vi "Add Annotation.vi"(8 "error in (no error)":errorcluster, 9 "Style":T1, 10 "Name":string, 11 "FSM.Edge in":refnum<class "FSM.Edge.lvclass">) -> (0 "error out":errorcluster, 2 "Changed?":bool, 3 "FSM.Edge out":refnum<class "FSM.Edge.lvclass">)   [LabVIEW 2015, in "FSM.Edge.lvclass"]
uses:
  FSM.Edge.lvclass
  FSM.Annotation/Annotation Style.ctl
  FSM.Edge.lvclass/FSM.Edge.ctl
  FSM.Annotation/FSM.Annotation.lvclass
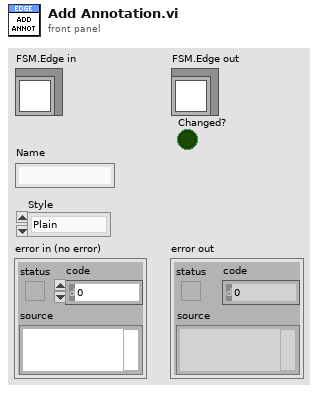
[diagram p1: front panel]
types:
  T1 = typedef "FSM.Annotation.lvclass/Annotation Style.ctl" = enum16{"Plain", "On", "Off", "On-Off"}
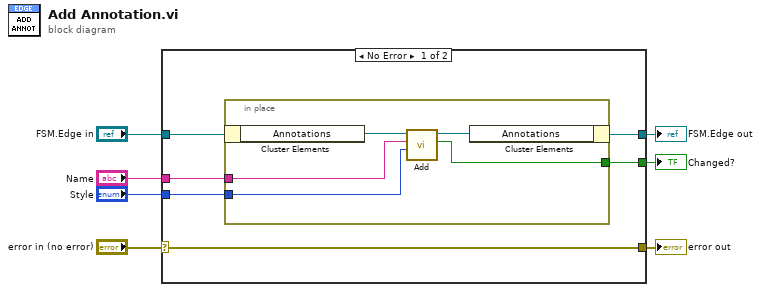
[diagram p0: block diagram]
diagram:
  n1 = case shown="No Error" "error in (no error)" {
    selector: "error in (no error)" -> [w13 w20]
    tunnel: [w13 w20] -> w6
    tunnel: [w9 w19] -> w4
    tunnel: "FSM.Edge in" -> [w10 w19]
    tunnel: "Name" -> [w11 _]
    tunnel: "Style" -> [w12 _]
    tunnel: [w8 _] -> w1
    frame No Error {
      n2 = in-place {
        in-place-border: w12 -> [w15]
        in-place-border: w11 -> [w16]
        in-place-border: [w14] -> w8
        n3 = in-place-cluster #1(w10) -> ("Annotations"=w18:refnum<class "FSM.Annotation.lvclass">)
        n4 = call "Add.vi"("Style"=w15, "Name"=w16, "FSM.Annotation in"=w18) -> ("Changed?"=w14:bool, "FSM.Annotation out"=w17:refnum<class "FSM.Annotation.lvclass">)  [unwired: 6 in, 1 out]
        n5 = in-place-cluster #1("Annotations"=w17) -> (w9:refnum<class "FSM.Edge.lvclass">)
      }
    }
    frame Error {
    }
  }
  "error out" <- w6
  "FSM.Edge out" <- w4
  "Changed?" <- w1
